vi "SetParam.vi"(8 "error in (no error)":errorcluster caption="entrée d'erreur (pas d'erreur)", 10 "fetch_california_housing":T1={"download_if_missing"=TRUE, "Returns"="Data"}, 11 "California_housing.lvclass":refnum<class "California_housing.lvclass">) -> (0 "error out":errorcluster caption="sortie d'erreur", 3 "California_housing.lvclass":refnum<class "California_housing.lvclass">)   [LabVIEW 2020, in "California_housing.lvclass"]
doc: "Set Parameters"
uses:
  California_housing.lvclass
  California_housing.lvclass/California_housing.ctl
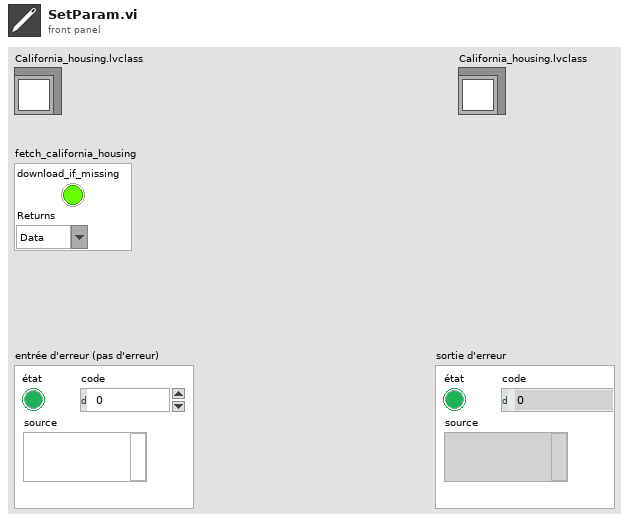
[diagram p1: front panel]
types:
  T1 = cluster{"download_if_missing":bool, "Returns":string}
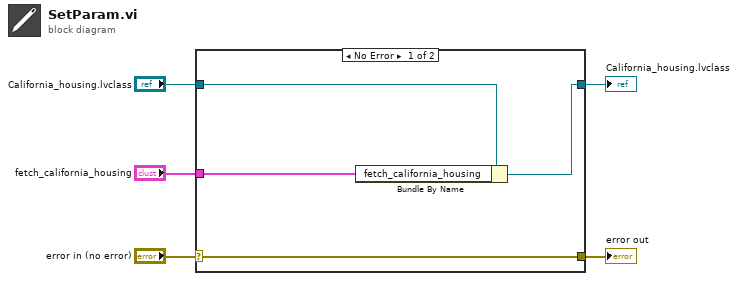
[diagram p0: block diagram]
diagram:
  n1 = case shown="No Error" "error in (no error)" {
    selector: "error in (no error)" -> [w9 w10]
    tunnel: [w9 w10] -> w4
    tunnel: [w7 w11] -> w2
    tunnel: "California_housing.lvclass" -> [w8 w11]
    tunnel: "fetch_california_housing" -> [w6 _]
    frame No Error {
      n2 = Bundle By Name(cluster=w8, "fetch_california_housing"=w6) -> (w7:refnum<class "California_housing.lvclass">)
    }
    frame Error {
    }
  }
  "error out" <- w4
  "California_housing.lvclass" <- w2
